vi "dfd_SCL_MAminm_CU.vi"(9 "global reset":bool, 11 "index":u16) -> (1 "control info":T1)   [LabVIEW 2017]
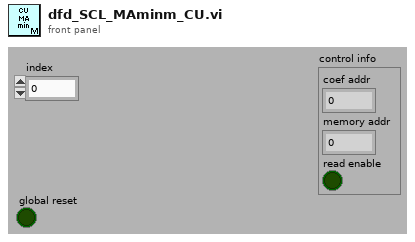
[diagram p1: front panel]
types:
  T1 = cluster{"coef addr":u16, "memory addr":u16, "read enable":bool}
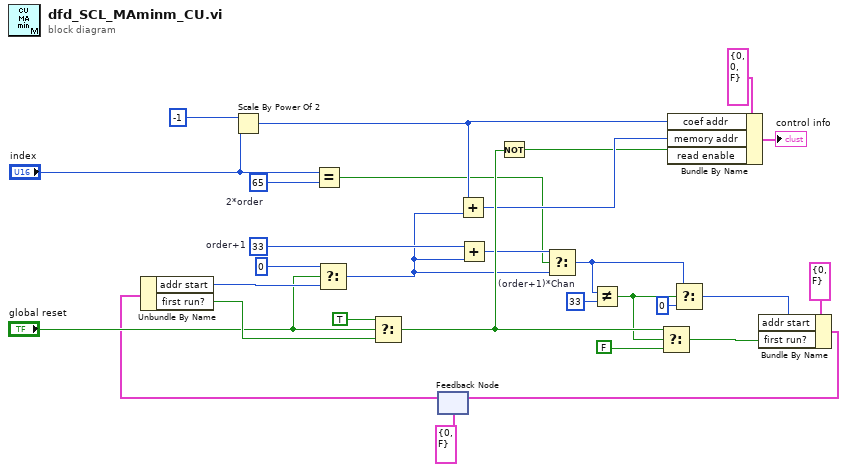
[diagram p0: block diagram]
diagram:
  w9 = u16 65  # 2*order
  w17 = u16 33  # (order+1)*Chan
  w21 = u16 33  # order+1
  n1 = Scale By Power Of 2(n=-1, x="index") -> (x*2^n=w8:u16)
  n2 = Equal?(x="index", y=w9) -> (x = y?=w7:bool)
  n3 = feedback #1(cluster{"addr start":u16, "first run?":bool} {"addr start"=0, "first run?"=FALSE} ("states")) -> (w3:cluster{"addr start":u16, "first run?":bool})
  n4 = Unbundle By Name(w3) -> ("addr start"=w28:u16, "first run?"=w29:bool)
  n5 = Select(t=u16 0, s="global reset", f=w28) -> (s? t:f=w5:u16)
  n6 = Select(t=TRUE, s="global reset", f=w29) -> (s? t:f=w26:bool)
  n7 = Add(x=w8, y=w5) -> (x+y=w14:u16)
  n8 = Add(x=w21, y=w5) -> (x+y=w19:u16)
  n9 = Not(x=w26) -> (.not. x?=w6:bool)
  n10 = Select(t=w19, s=w7, f=w5) -> (s? t:f=w20:u16)
  n11 = Not Equal?(x=w20, y=w17) -> (x != y?=w23:bool)
  n12 = Select(t=w26, s=w23, f=FALSE ("t")) -> (s? t:f=w27:bool)
  n13 = Bundle By Name(cluster=T1 {"coef addr"=0, "memory addr"=0, "read enable"=FALSE} ("control info 2"), "coef addr"=w8, "memory addr"=w14, "read enable"=w6) -> (→"control info":T1)
  n14 = Select(t=w20, s=w23, f=u16 0) -> (s? t:f=w15:u16)
  n15 = Bundle By Name(cluster=cluster{"addr start":u16, "first run?":bool} {"addr start"=0, "first run?"=FALSE} ("states"), "addr start"=w15, "first run?"=w27) -> (w4:cluster{"addr start":u16, "first run?":bool})
  n16 = feedback-in #1(w4) -> ()
